vi "vms_acceptCommand_start.vi"(8 "error in (no error)":errorcluster, 11 "command_start_Ctl":T1) -> (0 "error out":errorcluster, 2 "function return":i32, 3 "command_start_Ctl out":T1)   [LabVIEW 2016, in "SALLV_vms.lvlib"]
doc: "int vms_shm_acceptCommand_startLV(vms_command_startLV *command_start_Ctl );"
uses:
  SALLV_vms.lvlib
  DataTypes/command_start.ctl
  SALLV_vms.so
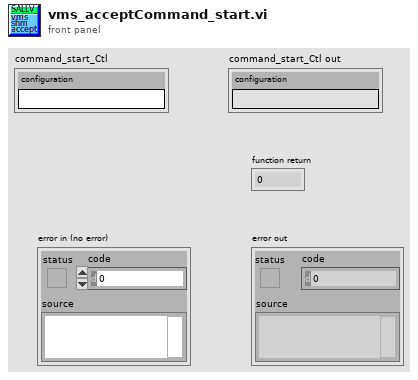
[diagram p1: front panel]
types:
  T1 = typedef "SALLV_vms.lvlib/command_start.ctl" = cluster{"configuration":string}
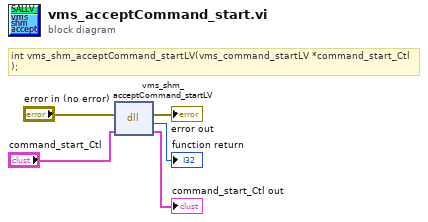
[diagram p0: block diagram]
diagram:
  # "int vms_shm_acceptCommand_startLV(vms_command_startLV *command_start_Ctl );"
  n1 = dll-call lib="opt/CODE/SALLV_vms/SALLV_vms.*" fn="vms_shm_acceptCommand_startLV"(error in="error in (no error)", "command_start_Ctl"="command_start_Ctl") -> (error out=→"error out":errorcluster, →"function return":i32, "command_start_Ctl"=→"command_start_Ctl out":T1)  [unwired: 2 in, 1 out]
